vi "lidar.vi"(8 "error in (no error)":errorcluster) -> (0 "error out":errorcluster, 2 "range Out":dbl[](array[numeric]), 3 "index Out":i32[](array[numeric]))   [LabVIEW 2018]
doc: "The myRIO Project template acquires acceleration data from the onboard accelerometer and displays the changes of acceleration values in a waveform chart."
uses:
  <vilib>/myRIO/Instrument Drivers/Onboard IO/UART/typedef/VISA Configuration.ctl
  <vilib>/Instr/_visa.llb/VISA Flush IO Buffer Mask.ctl
  <vilib>/Instr/_visa.llb/VISA Configure Serial Port (Instr).vi
  <vilib>/myRIO/Instrument Drivers/Onboard IO/UART/UART.lvlib
panel:
  in  "polar attributes":T1={"maximum"=100.0, "minimum"=0.0, "clip to min"=FALSE, "log?(F)"=FALSE, "grid color"=6710886, "plot color"=16711680, "fmt and prec"={"format"=enum."Decimal", "precision"=0}, "visible section"=8} {"minimum" format="%0.2f"; "maximum" format="%0.2f"}
  out "Lidar Data":picture
  out "range":dbl[](array[numeric])
  out "index":i32[](array[numeric])
  out "Boolean array":bool[](array[boolean])
  out "output array 2":bool[](array[boolean])
  out "Numeric Control":i32
  out "Character Count":u32
  in  "Characters to Write":string="b"
  out "Array":string[](array[string])
  out "read buffer 2":string
  out "read buffer":string
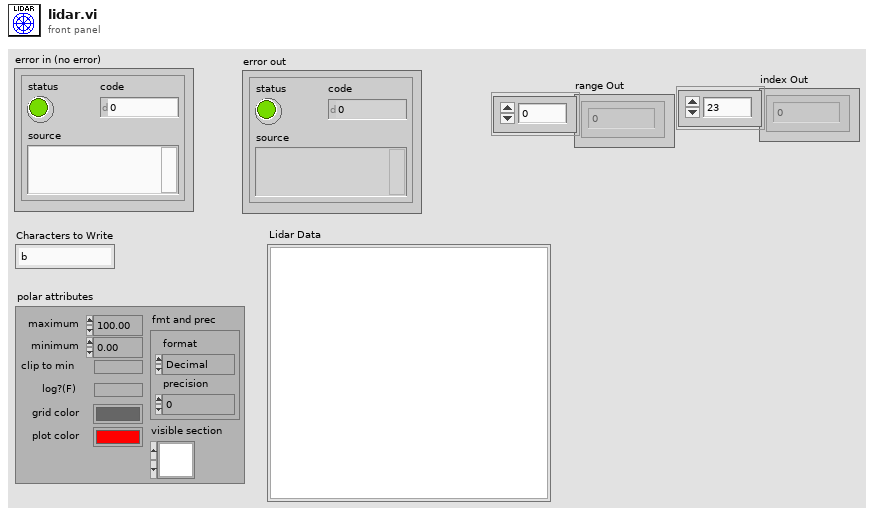
[diagram p1: front panel]
types:
  T1 = cluster{"maximum":dbl, "minimum":dbl, "clip to min":bool, "log?(F)":bool, "grid color":u32, "plot color":u32, "fmt and prec":cluster{"format":enum8{"Decimal", "Scientific", "Engineering", "Binary", "Octal", "Hex"}, "precision":u8}, "visible section":u16}
  T2 = typedef "VISA Flush IO Buffer Mask.ctl" = u16
  T3 = typedef "UART.lvlib/VISA Configuration.ctl" = cluster{"baud rate (9600)":u32, "data bits (8)":u16, "parity (0:none)":enum16{"None", "Odd", "Even", "Mark", "Space"}, "stop bits (10: 1 bit)":u16, "flow control (0:none)":u16, "termination char\n(0xA = '\\n' = LF) ":u8, "Enable Termination\nChar (T)":bool, "timeout (10sec)":u32}
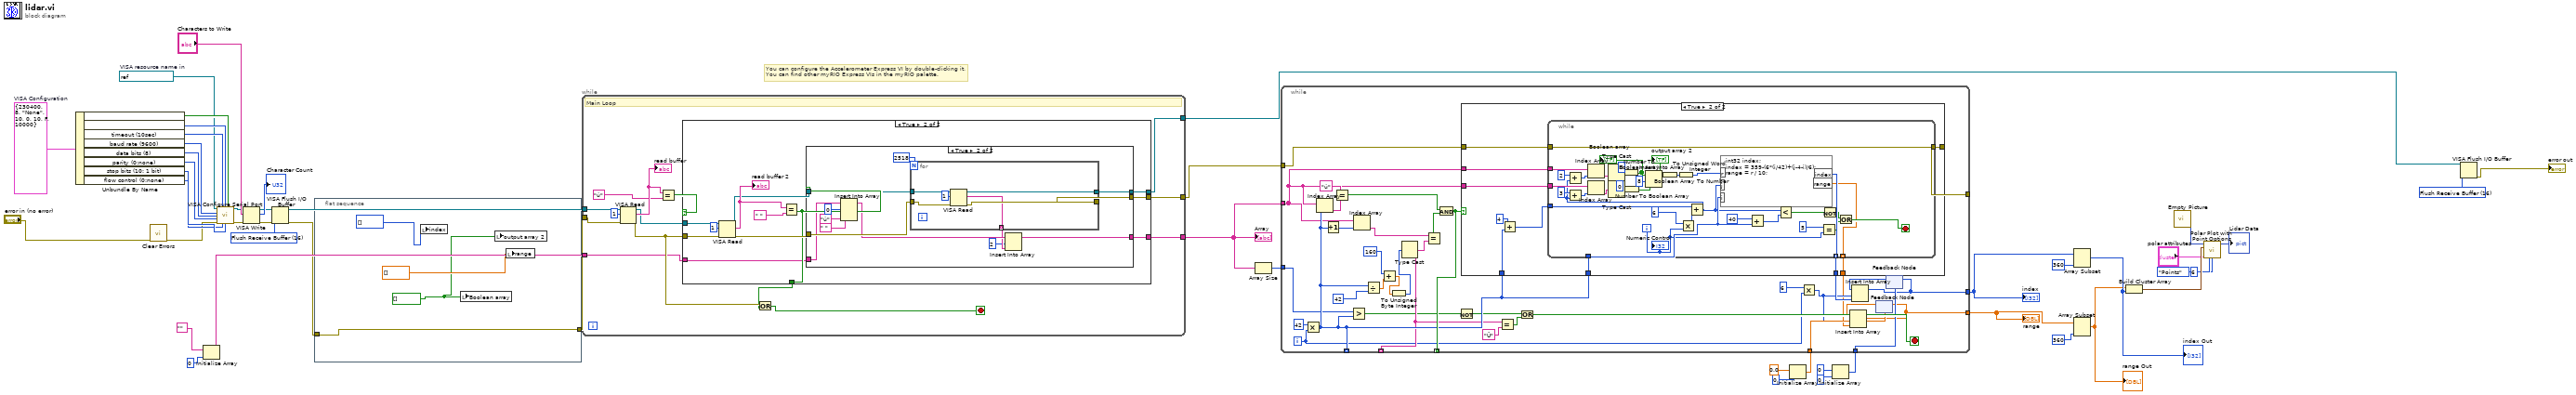
[diagram p0: block diagram]
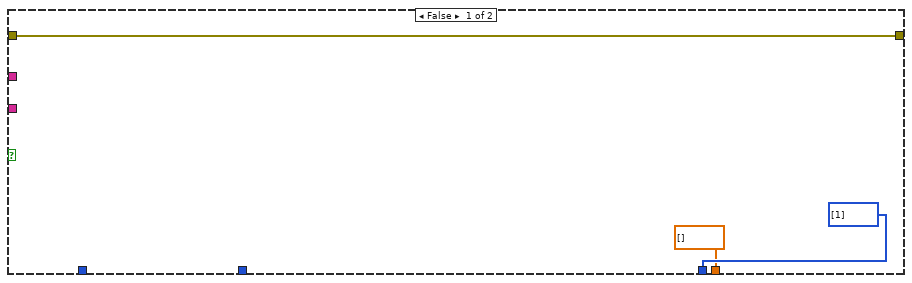
[diagram p2: hidden frame]
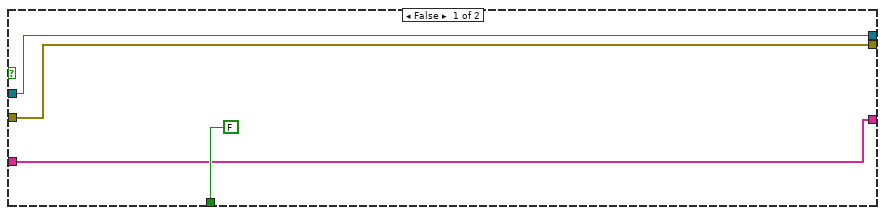
[diagram p3: hidden frame]
diagram:
  w19 = T2 16 items=["Flush Receive Buffer"=16, "Write Transmit Buffer to Device"=32, "Flush Receive Buffer (No I/O)"=64, "Flush Transmit Buffer"=128] ("Mask")
  w29 = T2 16 items=["Flush Receive Buffer"=16, "Write Transmit Buffer to Device"=32, "Flush Receive Buffer (No I/O)"=64, "Flush Transmit Buffer"=128] ("Mask")
  w49 = T3 {"baud rate (9600)"=230400, "data bits (8)"=8, "parity (0:none)"=enum."None", "stop bits (10: 1 bit)"=10, "flow control (0:none)"=0, "termination char\n(0xA = '\\n' = LF) "=10, "Enable Termination\nChar (T)"=FALSE, "timeout (10sec)"=10000}  # VISA Configuration
  w3 = refnum<visa-resource-name> "ASRL3::INSTR"  # VISA resource name in
  # "You can configure the Accelerometer Express VI by double-clicking it.\nYou can find other myRIO Express VIs in the myRIO palette."
  n1 = Unbundle By Name(w49) -> ("Enable Termination\nChar (T)"=w44:bool, "termination char\n(0xA = '\\n' = LF)"=w43:u8, "timeout (10sec)"=w42:u32, "baud rate (9600)"=w37:u32, "data bits (8)"=w38:u16, "parity (0:none)"=w39:enum16{"None", "Odd", "Even", "Mark", "Space"}, "stop bits (10: 1 bit)"=w40:u16, "flow control (0:none)"=w41:u16)
  n2 = call <vilib>:"Clear Errors.vi"("error in (no error)"="error in (no error)") -> ("error out"=w2:errorcluster)  [unwired: 5 in, 1 out]
  n3 = Initialize Array("", 0 ("dimension size")) -> (w34:string[])
  n4 = call-poly "VISA Configure Serial Port"("VISA resource name"=w3, "timeout (10sec)"=w42, "termination char\n(0xA = '\\n' = LF)"=w43, "Enable Termination\nChar (T)"=w44, "baud rate (9600)"=w37, "data bits (8)"=w38, "parity (0:none)"=w39, "error in (no error)"=w2, "stop bits (10: 1 bit)"=w40, "flow control (0:none)"=w41) -> ("VISA resource name out"=w46:refnum<visa-resource-name>, "error out"=w45:errorcluster)  [unwired: 4 in]
  n5 = VISA Write(VISA resource name=w46, write buffer="Characters to Write", error in (no error)=w45) -> (VISA resource name out=w30:refnum<visa-resource-name>, return count=→"Character Count":u32, error out=w31:errorcluster)
  n6 = VISA Flush I/O Buffer(VISA resource name=w30, mask (16)=w29, error in (no error)=w31) -> (VISA resource name out=w33:refnum<visa-resource-name>, error out=w32:errorcluster)
  n7 = flat-sequence {
    tunnel: w32 -> [w53]
    tunnel: [w53] -> w8
    frame #0 {
      w50 = bool[] []
      n8 = local write "index"(i32[] []) -> ()
      n9 = local write "Boolean array"(w50) -> ()
      n10 = local write "output array 2"(w50) -> ()
      n11 = local write "range"(dbl[] []) -> ()
    }
  }
  n12 = while {
    tunnel: [w63] -> w26
    tunnel: w33 -> [w58]
    tunnel: [w57] -> w27
    tunnel: w34 -> [w56]
    tunnel: [w55] -> w17
    tunnel: w8 -> [w54]
    stop <- w59 stop-if-true
    # "Main Loop"
    n13 = VISA Read(VISA resource name=w58, byte count=u32 1, error in (no error)=w54) -> (VISA resource name out=w64:refnum<visa-resource-name>, read buffer=w66:string, error out=w61:errorcluster)  [unwired: 1 out]
    "read buffer" <- w66
    n14 = Equal?(x=w66, y="ú") -> (x = y?=w62:bool)
    n15 = case shown="True" w62 {
      tunnel: w64 -> [w69 w82]
      tunnel: w61 -> [w70 w81]
      tunnel: [w70 w77] -> w63
      tunnel: [FALSE w75] -> w60
      tunnel: [w69 w74] -> w55
      tunnel: w56 -> [w68 w73]
      tunnel: [w68 w72] -> w57
      frame False {
      }
      frame True {
        n16 = VISA Read(VISA resource name=w82, byte count=u32 1, error in (no error)=w81) -> (VISA resource name out=w76:refnum<visa-resource-name>, read buffer=w79:string, error out=w78:errorcluster)  [unwired: 1 out]
        "read buffer 2" <- w79
        n17 = Equal?(x=w79, y=" ") -> (x = y?=w75:bool)
        n18 = case shown="True" w75 {
          tunnel: w78 -> [w86 w99]
          tunnel: [w86 w98] -> w77
          tunnel: w76 -> [w85 w96]
          tunnel: [w85 w95] -> w74
          tunnel: w73 -> [w84 w94]
          tunnel: [w84 w87] -> w72
          frame False {
          }
          frame True {
            n19 = Insert Into Array(array=w94, index=0, new element #1="ú" ("new element/subarray"), new element #2=" " ("new element/subarray")) -> (w90:string[])
            n20 = for {
              N: 2518 -> [_]
              tunnel: w99 -> [w104]
              tunnel: [w103] -> w98
              tunnel: [w102] -> w89 mode=indexing
              tunnel: w96 -> [w101]
              tunnel: [w100] -> w95
              n21 = VISA Read(VISA resource name=w101, byte count=u32 1, error in (no error)=w104) -> (VISA resource name out=w100:refnum<visa-resource-name>, read buffer=w102:string, error out=w103:errorcluster)  [unwired: 1 out]
            }
            n22 = Insert Into Array(array=w90, index=2, new element=w89) -> (w87:string[])
          }
        }
      }
    }
    n23 = Or(x=w61, y=w60) -> (x .or. y?=w59:bool)
  }
  "Array" <- w27
  n24 = Array Size(array=w27) -> (size(s)=w28:i32)
  n25 = Initialize Array(0.0, 0 ("dimension size")) -> (w20:dbl[])
  n26 = Initialize Array(0 ("element"), 0 ("dimension size")) -> (w25:i32[])
  n27 = while {
    tunnel: w28 -> [w124]
    tunnel: w27 -> [w111]
    tunnel: w26 -> [w133]
    tunnel: [w132] -> _
    tunnel: [w126] -> _ mode=indexing
    tunnel: [w122] -> _ mode=indexing
    tunnel: [w125] -> _ mode=indexing
    tunnel: w25 -> [w116]
    tunnel: [w112] -> w6
    tunnel: w20 -> [w109]
    tunnel: [w106] -> w7
    i -> [w115]
    stop <- w118 stop-if-true
    n28 = Multiply(x=42, y=w115) -> (x*y=w125:i32)
    n29 = Index Array(array=w111, index=w125) -> (element=w138:string)
    n30 = Increment(x=w125) -> (x+1=w137:i32)
    n31 = Equal?(x="ú", y=w138) -> (x = y?=w134:bool)
    n32 = Greater?(x=w124, y=w125) -> (0:w121:bool)
    n33 = Index Array(array=w111, index=w137) -> (element=w130:string)
    n34 = Divide(x=w125, y=42) -> (x/y=w129:dbl)
    n35 = Add(x=160 ("number"), y=w129) -> (x+y=w127:dbl)
    n36 = To Unsigned Byte Integer(number=w127) -> (unsigned 8bit integer=w128:u8)
    n37 = Type Cast(x=w128) -> (*(type *) &x=w122:string)  [unwired: 1 in]
    n38 = Equal?(x=w130, y=w122) -> (x = y?=w131:bool)
    n39 = And(x=w134, y=w131) -> (x .and. y?=w126:bool)
    n40 = Not(x=w121) -> (.not. x?=w119:bool)
    n41 = case shown="True" w126 {
      tunnel: w125 -> [_ w153]
      tunnel: w125 -> [_ w151]
      tunnel: w133 -> [w143 w149]
      tunnel: [w143 w148] -> w132
      tunnel: [i32[] [1] w147] -> w114
      tunnel: w111 -> [_ w146]
      tunnel: w111 -> [_ w145]
      tunnel: [dbl[] [] w144] -> w107
      frame False {
      }
      frame True {
        n42 = Add(x=4, y=w151) -> (x+y=w150:i32)
        n43 = while {
          tunnel: w153 -> [w181]
          tunnel: w150 -> [w186]
          tunnel: w149 -> [w180]
          tunnel: [w180] -> w148
          tunnel: [w179] -> w147 mode=indexing
          tunnel: w146 -> [w173]
          tunnel: w145 -> [w172]
          tunnel: [w154] -> w144 mode=indexing
          i -> [w175]
          stop <- w177 stop-if-true
          n44 = Multiply(x=6, y=w175) -> (x*y=w187:i32)
          n45 = Add(x=w186, y=w187) -> (x+y=w168:i32)
          n46 = Add(x=2, y=w168) -> (x+y=w169:i32)
          n47 = Add(x=3, y=w168) -> (x+y=w171:i32)
          n48 = Index Array(array=w172, index=w169) -> (element=w164:string)
          n49 = Index Array(array=w173, index=w171) -> (element=w161:string)
          n50 = Type Cast(type=u8 0, x=w164) -> (*(type *) &x=w166:u8)
          n51 = Type Cast(type=u8 0, x=w161) -> (*(type *) &x=w162:u8)
          n52 = Number To Boolean Array(number=w166) -> (Boolean array=w160:bool[])
          "Boolean array" <- w160
          n53 = Number To Boolean Array(number=w162) -> (Boolean array=w158:bool[])
          n54 = Insert Into Array(array=w160, index=8, new element=w158) -> (w157:bool[])
          "output array 2" <- w157
          n55 = Boolean Array To Number(Boolean array=w157) -> (number=w156:u32)
          n56 = To Unsigned Word Integer(number=w156) -> (unsigned 16bit integer=w155:u16)
          n57 = formula code="int32 index;\nindex = 359-(6*(i/42)+(j-4-i)/6);\nrange = r / 10;"("i"=w181, "j"=w168, "r"=w155) -> ("index"=w179:i32, "range"=w154:dbl)
          n58 = Add(x=40, y=w181) -> (x+y=w184:i32)
          n59 = Less?(x=w168, y=w184) -> (x < y?=w185:bool)
          n60 = Equal?(x=5, y=w175) -> (x = y?=w176:bool)
          n61 = Not(x=w185) -> (.not. x?=w178:bool)
          n62 = Or(x=w178, y=w176) -> (x .or. y?=w177:bool)
          "Numeric Control" <- w175
        }
      }
    }
    n63 = Equal?(x=w122, y="Û") -> (x = y?=w120:bool)
    n64 = Or(x=w119, y=w120) -> (x .or. y?=w118:bool)
    n65 = Multiply(x=6, y=w115) -> (x*y=w108:i32)
    n66 = feedback #1(w109) -> (w110:dbl[])
    n67 = Insert Into Array(array=w110, index=w108, new element=w107) -> (w106:dbl[])
    n68 = feedback-in #1(w106) -> ()
    n69 = feedback #2(w116) -> (w117:i32[])
    n70 = Insert Into Array(array=w117, index=w108, new element=w114) -> (w112:i32[])
    n71 = feedback-in #2(w112) -> ()
  }
  "index" <- w6
  "range" <- w7
  n72 = Array Subset(array=w6, length=360) -> (w5:i32[])  [unwired: 1 in]
  "index Out" <- w5
  n73 = Array Subset(array=w7, length=360) -> (w4:dbl[])  [unwired: 1 in]
  "range Out" <- w4
  n74 = Build Cluster Array(w4, w5) -> (w12:cluster{dbl, "element":i32}[])
  n75 = call "Empty Picture"() -> ("empty picture"=w14:picture)
  n76 = call <vilib>:"Polar Plot with Point Options.vi"("picture"=w14, "data array [mag, phase (deg)]"=w12, "polar attributes"="polar attributes", "Lines/Points"=enum16{"Lines", "Points"}."Points", "Size"=u16 6) -> ("new picture"=→"Lidar Data":picture)  [unwired: 10 in]
  n77 = VISA Flush I/O Buffer(VISA resource name=w17, mask (16)=w19) -> (error out=→"error out":errorcluster)  [unwired: 1 in, 1 out]
